vi "LogData.vi"(0 "file size":i64, 5 "File path":path, 7 "Numeric":dbl, 11 "Error in":errorcluster) -> (15 "Error out":errorcluster)   [LabVIEW 2020]
doc: "This VI is used to log the data which is generated by the generate VI along with time the user can specify the size upto which data can be logged if the sixe exceeds error will be reported and execution will be stopped"
panel:
  # "Select the file to log thedata"
  # "Specify the size limit of the file"
  # "Data to be logged has to be wired"
  # "INPUT"
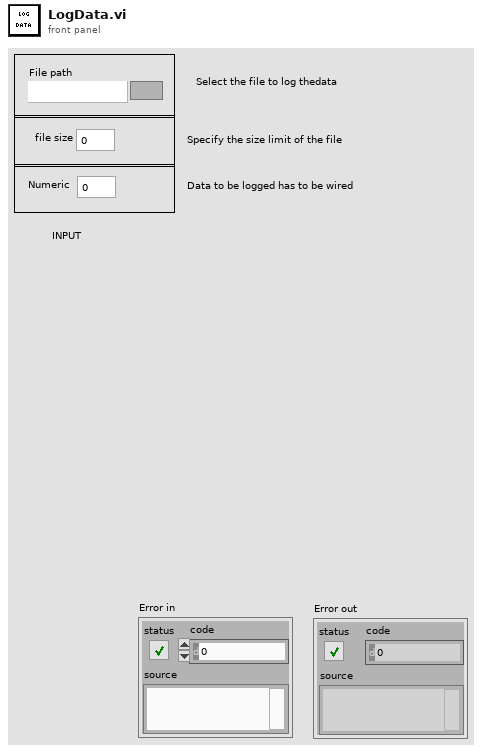
[diagram p1: front panel]
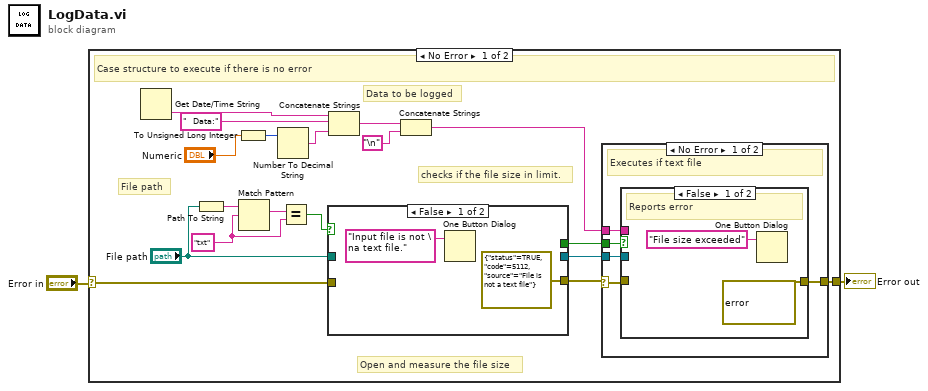
[diagram p0: block diagram]
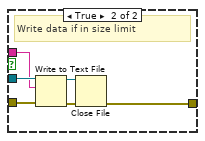
[diagram p2: hidden frame]
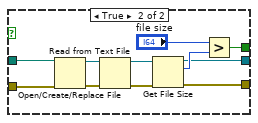
[diagram p4: hidden frame]
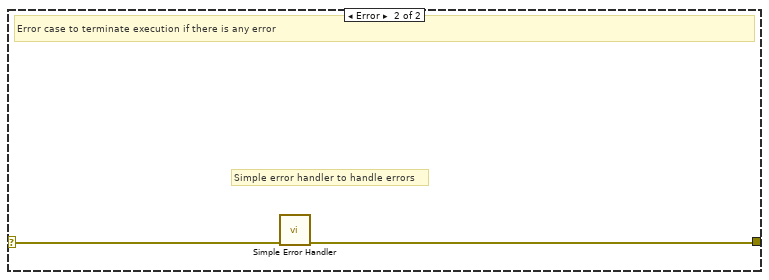
[diagram p5: hidden frame]
diagram:
  n1 = case shown="No Error" "Error in" {
    selector: "Error in" -> [w9 w49]
    tunnel: [w20 w48] -> w1
    frame No Error {
      w5 = "txt" ("regular expression")
      # "Data to be logged"
      # "File path"
      # "checks if the file size in limit."
      # "Open and measure the file size"
      # "Case structure to execute if there is no error"
      n2 = Get Date/Time String() -> (time string=w17:string)  [unwired: 3 in, 1 out]
      n3 = Path To String(path="File path") -> (string=w8:string)
      n4 = To Unsigned Long Integer(number="Numeric") -> (unsigned 32bit integer=w11:u32)
      n5 = Match Pattern(string=w8, regular expression=w5) -> (match substring=w6:string)  [unwired: 1 in, 3 out]
      n6 = Number To Decimal String(number=w11) -> (decimal integer string=w19:string)  [unwired: 1 in]
      n7 = Equal?(x=w6, y=w5) -> (x = y?=w4:bool)
      n8 = case shown="False" w4 {
        tunnel: [_ w41] -> w14
        tunnel: [errorcluster {"status"=TRUE, "code"=5112, "source"="File is not a text file"} ("error out") w40] -> w3
        tunnel: [_ w39] -> w13
        tunnel: w9 -> [_ w38]
        tunnel: "File path" -> [_ w37]
        frame False {
          n9 = One Button Dialog(message="Input file is not \na text file.") -> ()  [unwired: 1 in, 1 out]
        }
        frame True {
          n10 = Open/Create/Replace File(file path (use dialog)=w37, error in=w38) -> (refnum out=w46:refnum<file>, error out=w47:errorcluster)  [unwired: 4 in, 1 out]
          n11 = Read from Text File(file (use dialog)=w46, error in=w47) -> (refnum out=w44:refnum<file>, error out=w45:errorcluster)  [unwired: 2 in, 2 out]
          n12 = Get File Size(file=w44, error in=w45) -> (refnum out=w39:refnum<file>, size (in bytes)=w43:i64, 0:w40:errorcluster)
          n13 = Greater?(x="file size", y=w43) -> (0:w41:bool)
        }
      }
      n14 = Concatenate Strings(w17, "  Data:" ("string"), w19) -> (w18:string)
      n15 = Concatenate Strings(w18, "\n") -> (w12:string)
      n16 = case shown="No Error" w3 {
        selector: w3 -> [w21 w34]
        tunnel: [w25 w34] -> w20
        tunnel: w14 -> [w24 _]
        tunnel: w13 -> [w23 _]
        tunnel: w12 -> [w22 _]
        frame No Error {
          # "Executes if text file"
          n17 = case shown="False" w24 {
            tunnel: [errorcluster {"status"=TRUE, "code"=5129, "source"="The file size exceeds the \noperable limit no data will be logged further.\nLocation:Storagefile\\Log.txt\n"} ("error out") w31] -> w25
            tunnel: w21 -> [_ w30]
            tunnel: w23 -> [_ w29]
            tunnel: w22 -> [_ w28]
            frame False {
              # "Reports error"
              n18 = One Button Dialog(message="File size exceeded") -> ()  [unwired: 1 in, 1 out]
            }
            frame True {
              # "Write data if in size limit"
              n19 = Write to Text File(file (use dialog)=w29, text=w28, error in=w30) -> (refnum out=w32:refnum<file>, error out=w33:errorcluster)  [unwired: 1 in, 1 out]
              n20 = Close File(refnum=w32, error in=w33) -> (error out=w31:errorcluster)  [unwired: 1 out]
            }
          }
        }
        frame Error {
          # "Reports error if file\nis not a text file"
        }
      }
    }
    frame Error {
      # "Simple error handler to handle errors"
      # "Error case to terminate execution if there is any error"
      n21 = call <vilib>:"Simple Error Handler.vi"("error in (no error)"=w49) -> ("error out"=w48:errorcluster)  [unwired: 4 in, 4 out]
    }
  }
  "Error out" <- w1
